vi "Disable Source Separation.vi"(9 "Operation Start Time":timestamp, 11 "Root Path":path) -> ()   [LabVIEW 2014]
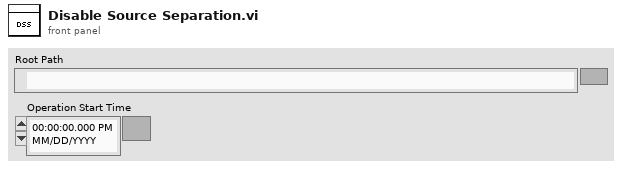
[diagram p1: front panel]
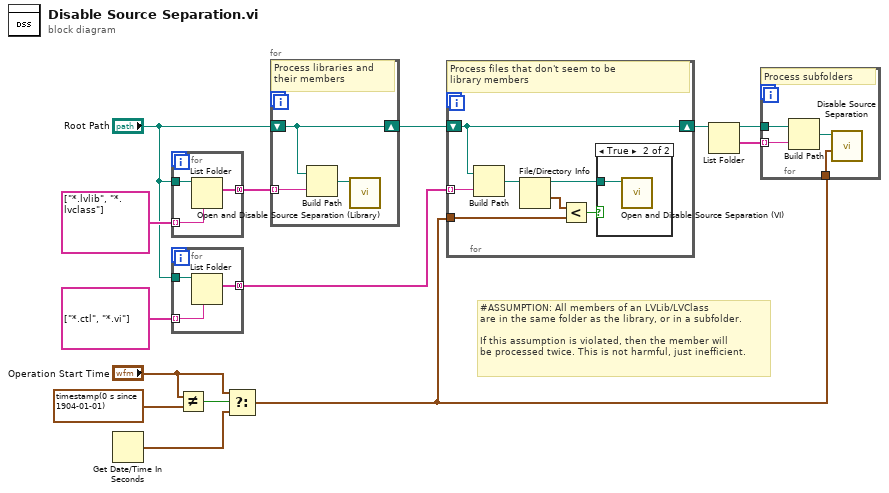
[diagram p0: block diagram]
diagram:
  # "#ASSUMPTION: All members of an LVLib/LVClass\nare in the same folder as the library, or in a subfolder.\n\nIf this assumption is violated, then the member will\nbe processed twice. This is not harmful, just inefficient."
  n1 = Get Date/Time In Seconds() -> (seconds since 1Jan1904=w6:timestamp)
  n2 = for {
    tunnel: "Root Path" -> [w17]
    tunnel: [w16] -> w13 mode=concatenating
    tunnel: string[] ["*.lvlib", "*.lvclass"] -> [w15] mode=indexing
    n3 = List Folder(path=w17, pattern=w15) -> (filenames=w16:string[])  [unwired: 2 in, 3 out]
  }
  n4 = for {
    tunnel: "Root Path" -> [w20]
    tunnel: [w19] -> w10 mode=concatenating
    tunnel: string[] ["*.ctl", "*.vi"] -> [w18] mode=indexing
    n5 = List Folder(path=w20, pattern=w18) -> (filenames=w19:string[])  [unwired: 2 in, 3 out]
  }
  n6 = Not Equal?(x="Operation Start Time", y=timestamp(0 s since 1904-01-01)) -> (x != y?=w8:bool)
  n7 = Select(t="Operation Start Time", s=w8, f=w6) -> (s? t:f=w1:timestamp)
  n8 = for {
    tunnel: w13 -> [w23] mode=indexing
    shift-right: [w21] -> w3
    shift-left: "Root Path" -> [w21]
    # "Process libraries and\ntheir members"
    n9 = Build Path(base path=w21, name or relative path=w23) -> (appended path=w22:path)
    n10 = call "Open and Disable Source Separation (Library).vi"("Library Path"=w22) -> ()  [unwired: 11 in]
  }
  n11 = for {
    tunnel: w10 -> [w30] mode=indexing
    tunnel: w1 -> [w29]
    shift-right: [w24] -> w2
    shift-left: w3 -> [w24]
    # "Process files that don't seem to be\nlibrary members"
    n12 = Build Path(base path=w24, name or relative path=w30) -> (appended path=w28:path)
    n13 = File/Directory Info(path=w28) -> (path out=w25:path, last mod=w27:timestamp)  [unwired: 1 in, 5 out]
    n14 = Less?(x=w27, y=w29) -> (x < y?=w26:bool)
    n15 = case shown="True" w26 {
      tunnel: w25 -> [_ w31]
      frame False {
      }
      frame True {
        n16 = call "Open and Disable Source Separation (VI).vi"("VI Path"=w31) -> ()  [unwired: 11 in]
      }
    }
  }
  n17 = List Folder(path=w2) -> (path out=w5:path, folder names=w4:string[])  [unwired: 3 in, 2 out]
  n18 = for {
    tunnel: w5 -> [w35]
    tunnel: w4 -> [w34] mode=indexing
    tunnel: w1 -> [w32]
    # "Process subfolders"
    n19 = Build Path(base path=w35, name or relative path=w34) -> (appended path=w33:path)
    n20 = call "Disable Source Separation.vi"("Operation Start Time"=w32, "Root Path"=w33) -> ()  [unwired: 10 in]
  }
